vi "PSTR-Load Data.vi"(7 "selected path":path, 11 "error in (no error)":errorcluster, 12 "check":bool=TRUE) -> (4 "Params":T6={"Stimulus"={"Ear"=enum."Right", "BW (oct)"=0.3333, "Seed"=37, "Ramp (ms)"=1.0, "On time (ms)"=200.0, "Off time (ms)"=200.0, "Delay (ms)"=0.0}, "FreqSeq"={"Min (kHz)"=2.0, "Max (kHz)"=2.0, "Step (oct)"=0.5}, "LevelSeq"={"Min (dB)"=0.0, "Max (dB)"=80.0, "Step (dB)"=10.0}, "Seq"={"Order"=enum."Sequential", "Averages"=50}, "Response"={"Grass gain"=10000.0, "Window (ms)"=200.0}, "Hidden"={"Sample rate (Hz)"=100000.0, "Nfft"=2048, "save raw"=TRUE, "sep"=0.0, "Window"=enum."NONE"}, "RejThr"=0.0}, 6 "Data":T3, 8 "CFTS-PSTR":T2, 15 "error out":errorcluster)   [LabVIEW 2020]
uses:
  Typedefs/PSTR-Parameters.ctl
  Typedefs/PSTR-Stimulus Params.ctl
  epl-vi-lib/Utility VIs/Type Defs/Left-Right ring.ctl
  Typedefs/PSTR-FreqSeq Params.ctl
  Typedefs/PSTR-LevelSeq Params.ctl
  Typedefs/PSTR-SeqParams.ctl
  Typedefs/PSTR-Response Params.ctl
  Typedefs/PSTR-Hidden Params.ctl
  Typedefs/PSTR-Window Shape.ctl
  Typedefs/PSTR-Data.ctl
  Typedefs/PSTR-Model Fit.ctl
  Typedefs/PSTR-Fit Parameters.ctl
  Typedefs/PSTR-File Info.ctl
  <vilib>/regexp/Match Regular Expression.xnode
panel:
  in  "Data":T1
  # "NF x NL x 2 x Npts"
  # "NF x NL x Npts"
  # "NF x NL"
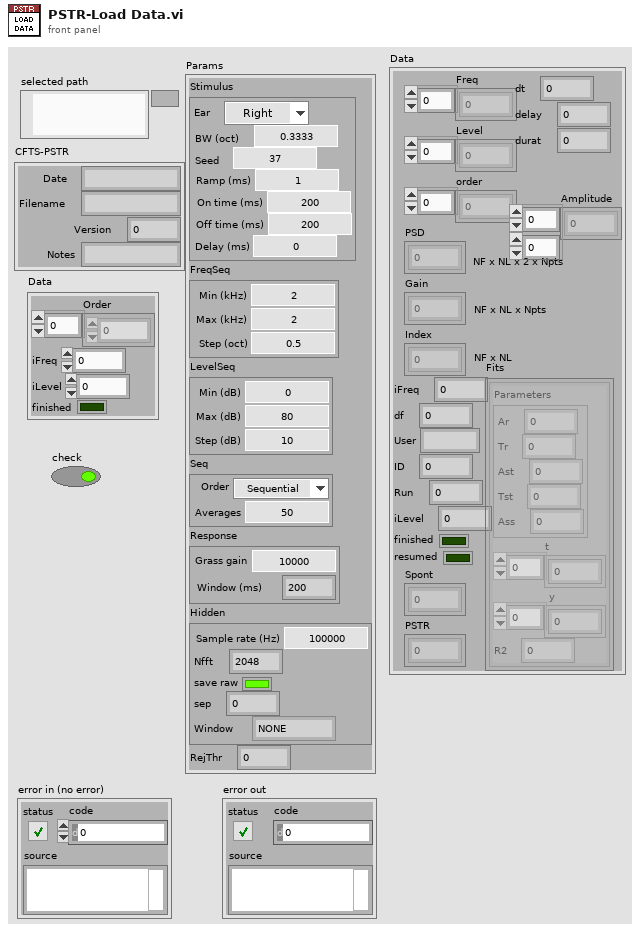
[diagram p1: front panel]
types:
  T1 = cluster{"Order":i32[], "iFreq":i32, "iLevel":i32, "finished":bool}
  T2 = typedef "PSTR-File Info.ctl" = cluster{"Date":string, "Filename":string, "Version":i32, "Notes":string}
  T3 = typedef "PSTR-Data.ctl" = cluster{"Freq":dbl[], "Level":dbl[], "order":i32[], "PSD":dbl[][][][], "Gain":dbl[][][], "Index":dbl[][], "iFreq":i32, "df":dbl, "User":string, "ID":i32, "Run":i32, "iLevel":i32, "finished":bool, "resumed":bool, "Spont":dbl[][], "PSTR":dbl[][][], "dt":dbl, "delay":dbl, "durat":dbl, "Fits":T4[][], "Amplitude":dbl[][]}
  T4 = typedef "PSTR-Model Fit.ctl" = cluster{"Parameters":T5, "t":dbl[], "y":dbl[], "R2":dbl}
  T5 = typedef "PSTR-Fit Parameters.ctl" = cluster{"Ar":dbl, "Tr":dbl, "Ast":dbl, "Tst":dbl, "Ass":dbl}
  T6 = typedef "PSTR-Parameters.ctl" = cluster{"Stimulus":T7, "FreqSeq":T9, "LevelSeq":T10, "Seq":T11, "Response":T12, "Hidden":T13, "RejThr":dbl}
  T7 = typedef "PSTR-Stimulus Params.ctl" = cluster{"Ear":T8, "BW (oct)":dbl, "Seed":i32, "Ramp (ms)":dbl, "On time (ms)":dbl, "Off time (ms)":dbl, "Delay (ms)":dbl}
  T8 = typedef "Left-Right ring.ctl" = enum16{"Right", "Left"}
  T9 = typedef "PSTR-FreqSeq Params.ctl" = cluster{"Min (kHz)":dbl, "Max (kHz)":dbl, "Step (oct)":dbl}
  T10 = typedef "PSTR-LevelSeq Params.ctl" = cluster{"Min (dB)":dbl, "Max (dB)":dbl, "Step (dB)":dbl}
  T11 = typedef "PSTR-SeqParams.ctl" = cluster{"Order":enum16{"Sequential", "Random"}, "Averages":i32}
  T12 = typedef "PSTR-Response Params.ctl" = cluster{"Grass gain":dbl, "Window (ms)":dbl}
  T13 = typedef "PSTR-Hidden Params.ctl" = cluster{"Sample rate (Hz)":dbl, "Nfft":i32, "save raw":bool, "sep":dbl, "Window":T14}
  T14 = typedef "PSTR-Window Shape.ctl" = enum16{"NONE", "Hamming"}
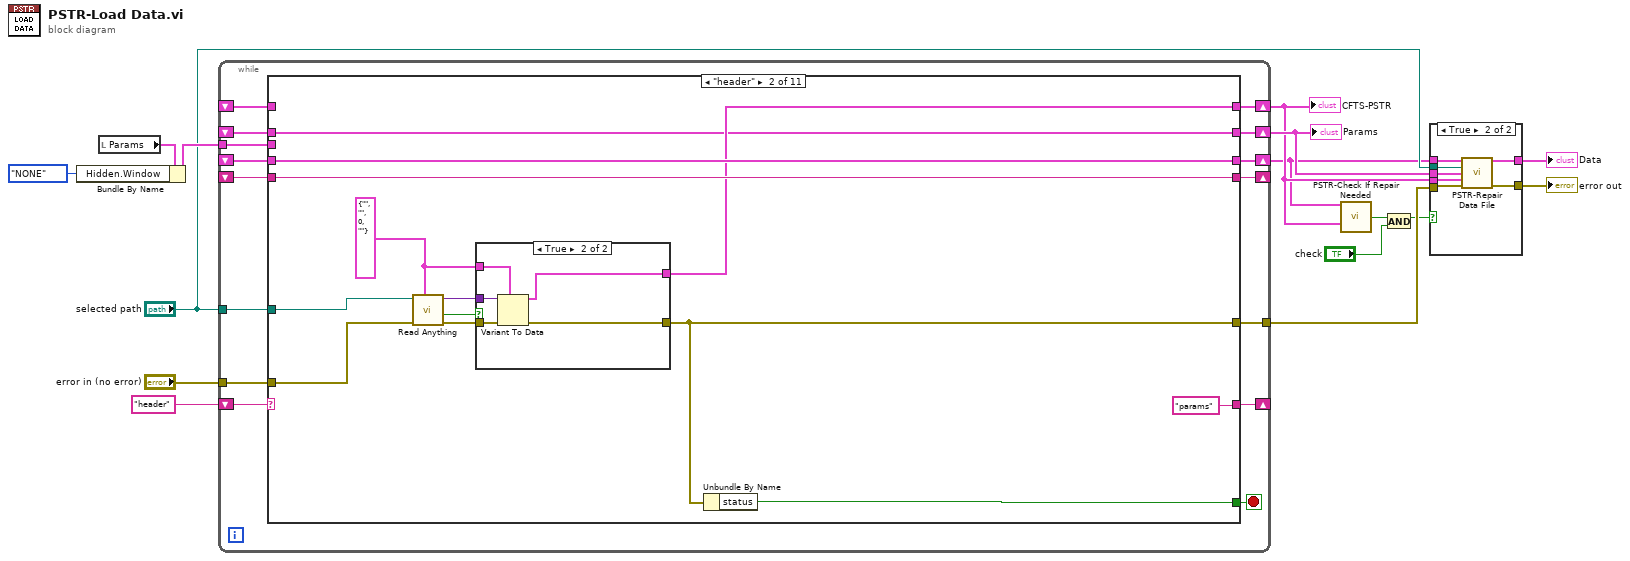
[diagram p0: block diagram]
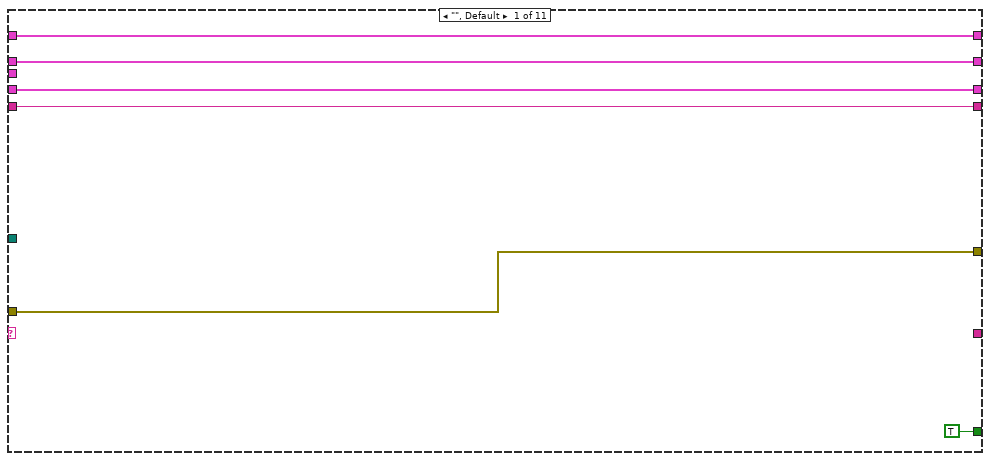
[diagram p2: hidden frame]
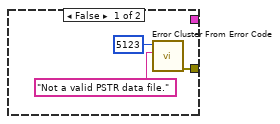
[diagram p3: hidden frame]
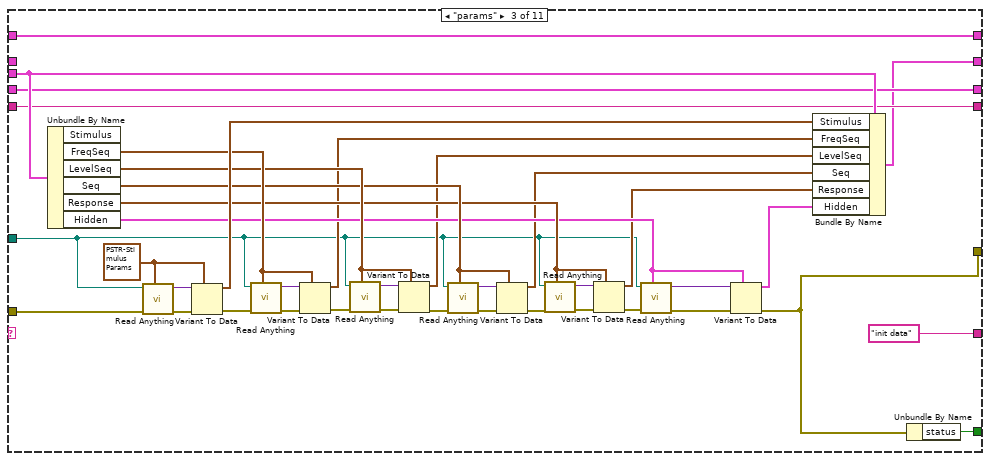
[diagram p4: hidden frame]
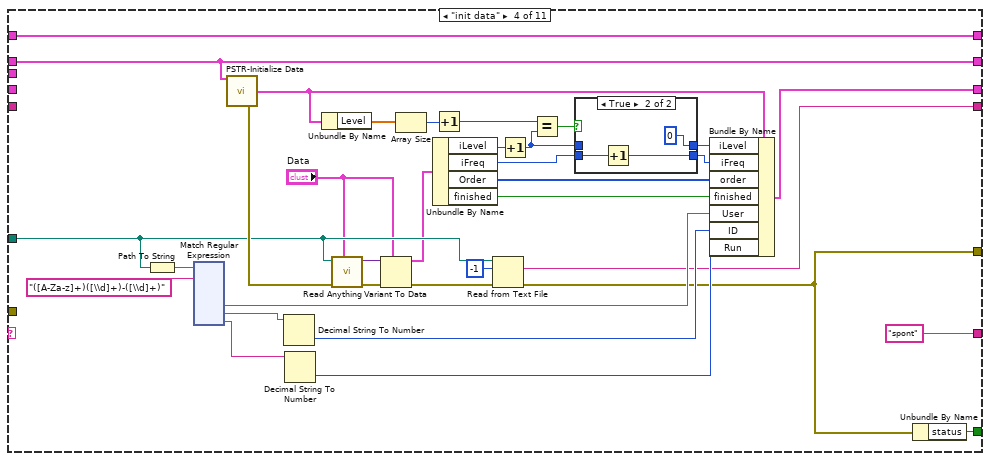
[diagram p5: hidden frame]
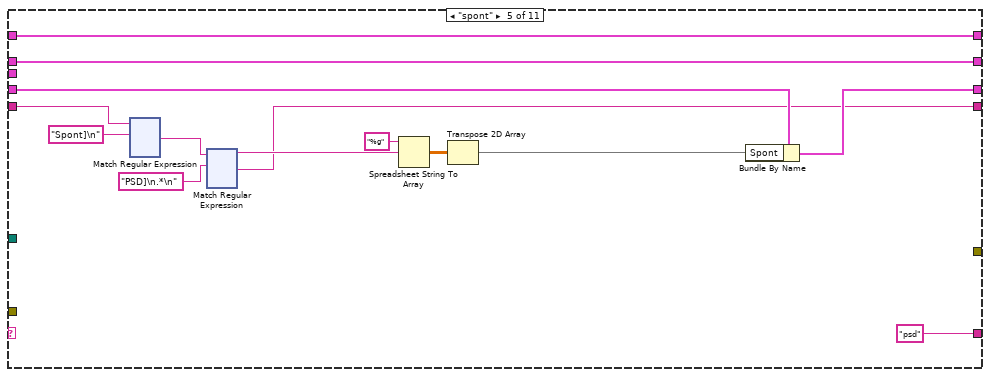
[diagram p7: hidden frame]
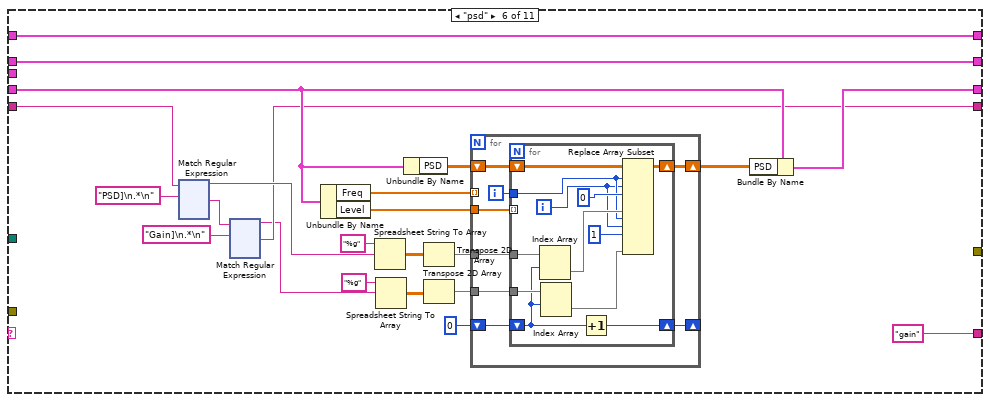
[diagram p8: hidden frame]
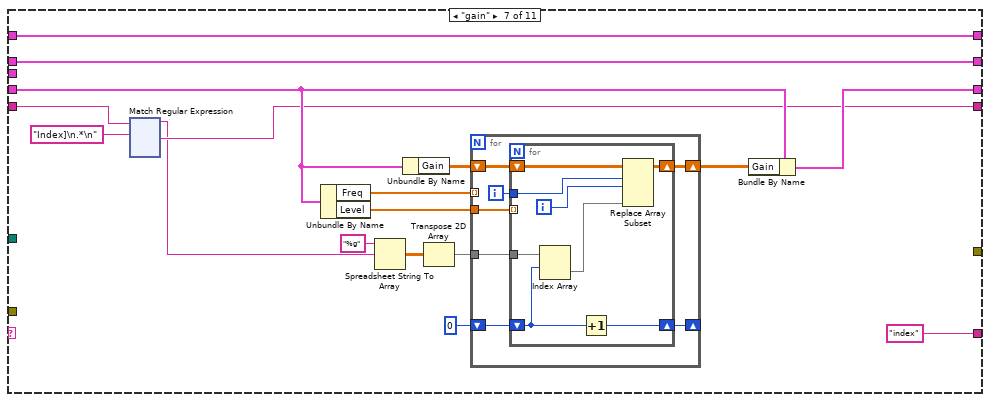
[diagram p9: hidden frame]
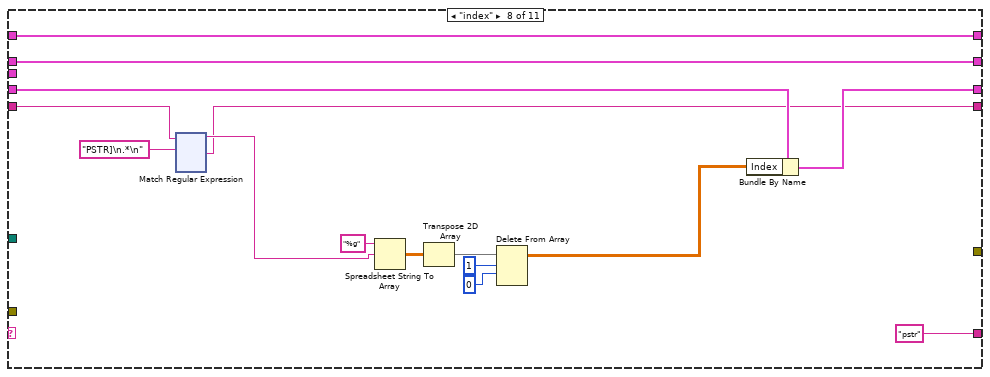
[diagram p10: hidden frame]
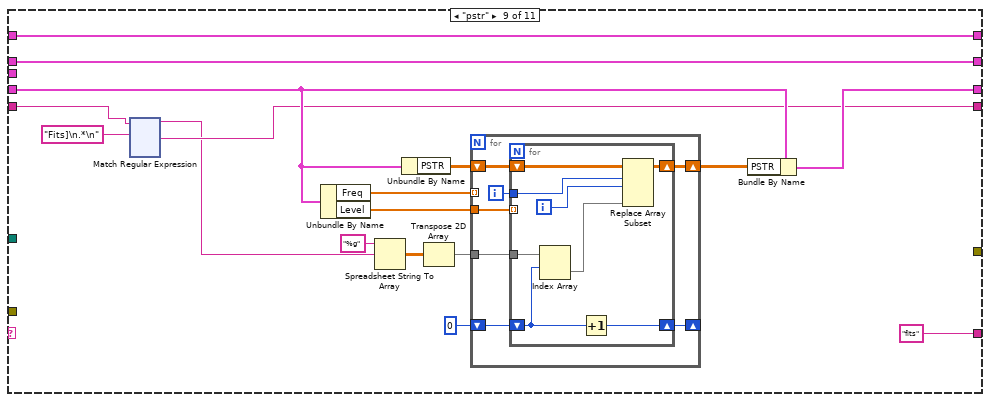
[diagram p11: hidden frame]
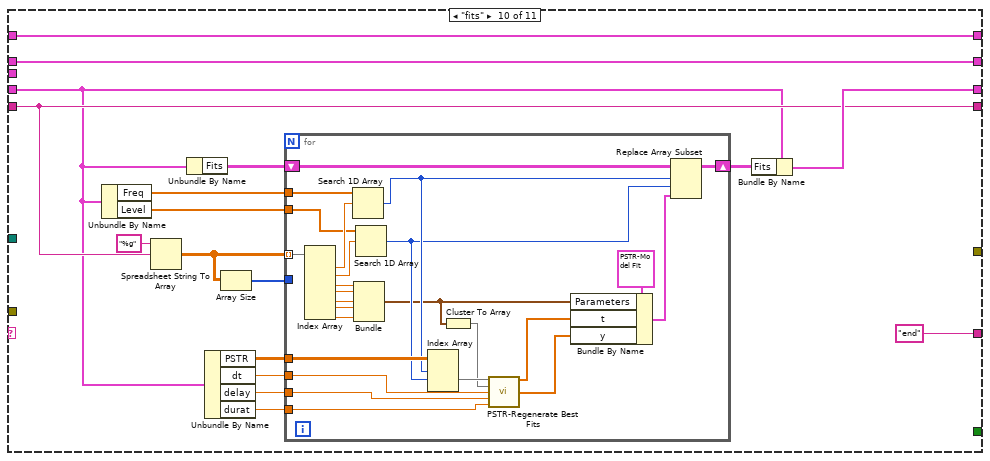
[diagram p12: hidden frame]
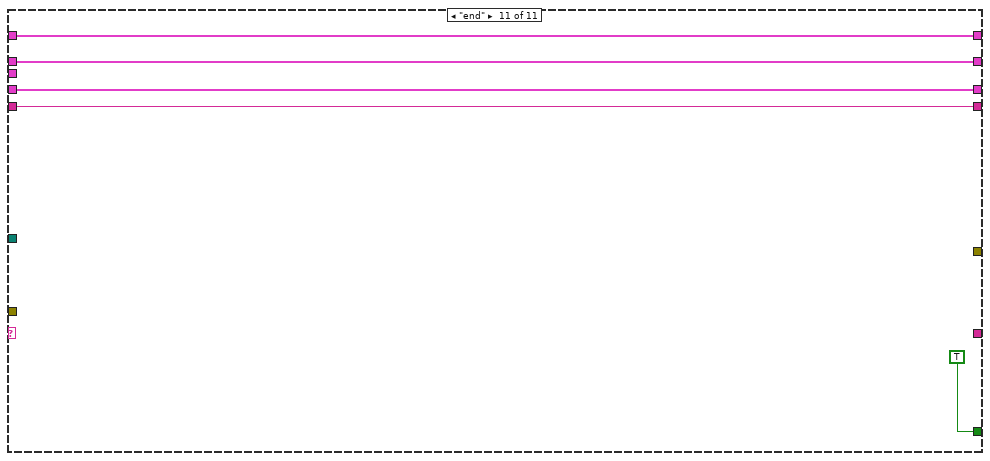
[diagram p13: hidden frame]
diagram:
  n1 = local read "Params"() -> (w13:T6)
  n2 = Bundle By Name(cluster=w13, "Hidden.Window"=PSTR-Window_Shape."NONE") -> (w12:T6)
  n3 = while {
    tunnel: "error in (no error)" -> [w30]
    tunnel: "selected path" -> [w29]
    shift-right: [w26] -> _
    shift-left: "header" -> [w28]
    tunnel: [w25] -> w3
    tunnel: w12 -> [w24]
    shift-right: [w23] -> w5
    shift-left: _ -> [w22]
    shift-right: [w21] -> _
    shift-left: _ -> [w20]
    shift-right: [w19] -> w6
    shift-left: _ -> [w18]
    shift-right: [w17] -> w8
    shift-left: _ -> [w16]
    stop <- w27 stop-if-true
    n4 = case shown="\"header\"" w28 {
      tunnel: w30 -> [w36 w49 w96 _ _ _ _ _ _ _ _]
      tunnel: w29 -> [_ w48 w63 w117 _ _ _ _ _ _ _]
      tunnel: [TRUE ("status") w42 w70 w126 _ _ _ _ _ _ TRUE ("status")] -> w27
      tunnel: [w36 w43 w71 w115 _ _ _ _ _ _ _] -> w25
      tunnel: [_ "params" "init data" "spont" "psd" "gain" "index" "pstr" "fits" "end" _] -> w26
      tunnel: w24 -> [_ _ w93 _ _ _ _ _ _ _ _]
      tunnel: [w34 w41 w62 w112 w265 w512 w777 w926 w1052 w1204 w1233] -> w23
      tunnel: w22 -> [w34 w41 w62 _ w266 w513 w778 w927 w1053 w1196 w1233]
      tunnel: [w33 w40 w61 w114 w256 w501 w770 w915 w1046 w1201 w1234] -> w21
      tunnel: w20 -> [w33 w40 w61 _ w263 w498 w773 w917 w1044 w1201 w1234]
      tunnel: [w32 w39 w59 w98 w255 w497 w768 w914 w1043 w1189 w1231] -> w19
      tunnel: w18 -> [w32 _ w59 w98 w255 w497 w768 w914 w1043 w1189 w1231]
      tunnel: [w31 w38 w58 w97 w254 w496 w767 w913 w1042 w1188 w1230] -> w17
      tunnel: w16 -> [w31 w38 _ w97 w254 w496 w767 w913 w1042 w1188 w1230]
      frame "", Default {
      }
      frame "header" {
        w37 = T2 {"Date"="", "Filename"="", "Version"=0, "Notes"=""} ("CFTS-PSTR")
        n5 = call "Read Anything.vi"("Type of Anything"=w37, "Error In"=w49, "Path (dialog)"=w48) -> ("Error Out"=w47:errorcluster, "Found?"=w46:bool, "Anything"=w45:variant)  [unwired: 6 in]
        n6 = case shown="True" w46 {
          tunnel: w47 -> [_ w57]
          tunnel: w45 -> [_ w56]
          tunnel: w37 -> [_ w55]
          tunnel: [w52 w54] -> w43
          tunnel: [_ w53] -> w39
          frame False {
            n7 = call <vilib>:"Error Cluster From Error Code.vi"("error message (\"\")"="Not a valid PSTR data file." ("error message (\"\")"), "error code (0)"=5123) -> ("error out"=w52:errorcluster)  [unwired: 7 in]
          }
          frame True {
            n8 = Variant To Data(error in=w57, type=w55, Variant=w56) -> (data=w53:T2, error out=w54:errorcluster)
          }
        }
        n9 = Unbundle By Name(w43) -> ("status"=w42:bool)
      }
      frame "params" {
        w60 = T7 {"Ear"=enum."Right", "BW (oct)"=0.25, "Seed"=37, "Ramp (ms)"=5.0, "On time (ms)"=300.0, "Off time (ms)"=300.0, "Delay (ms)"=0.0} ("Stimulus")
        n10 = Unbundle By Name(w93) -> ("FreqSeq"=w88:T9, "LevelSeq"=w84:T10, "Seq"=w74:T11, "Response"=w73:T12, "Hidden"=w72:T13)  [unwired: 1 out]
        n11 = call "Read Anything.vi"("Type of Anything"=w60, "Error In"=w96, "Path (dialog)"=w63) -> ("Error Out"=w95:errorcluster, "Anything"=w94:variant)  [unwired: 6 in, 1 out]
        n12 = Variant To Data(error in=w95, type=w60, Variant=w94) -> (data=w92:T7, error out=w89:errorcluster)
        n13 = call "Read Anything.vi"("Type of Anything"=w88, "Error In"=w89, "Path (dialog)"=w63) -> ("Error Out"=w91:errorcluster, "Anything"=w90:variant)  [unwired: 6 in, 1 out]
        n14 = Variant To Data(error in=w91, type=w88, Variant=w90) -> (data=w68:T9, error out=w86:errorcluster)
        n15 = call "Read Anything.vi"("Type of Anything"=w84, "Error In"=w86, "Path (dialog)"=w63) -> ("Error Out"=w87:errorcluster, "Anything"=w85:variant)  [unwired: 6 in, 1 out]
        n16 = Variant To Data(error in=w87, type=w84, Variant=w85) -> (data=w67:T10, error out=w77:errorcluster)
        n17 = call "Read Anything.vi"("Type of Anything"=w74, "Error In"=w77, "Path (dialog)"=w63) -> ("Error Out"=w83:errorcluster, "Anything"=w82:variant)  [unwired: 6 in, 1 out]
        n18 = Variant To Data(error in=w83, type=w74, Variant=w82) -> (data=w66:T11, error out=w76:errorcluster)
        n19 = call "Read Anything.vi"("Type of Anything"=w73, "Error In"=w76, "Path (dialog)"=w63) -> ("Error Out"=w81:errorcluster, "Anything"=w80:variant)  [unwired: 6 in, 1 out]
        n20 = Variant To Data(error in=w81, type=w73, Variant=w80) -> (data=w65:T12, error out=w75:errorcluster)
        n21 = call "Read Anything.vi"("Type of Anything"=w72, "Error In"=w75, "Path (dialog)"=w63) -> ("Error Out"=w79:errorcluster, "Anything"=w78:variant)  [unwired: 6 in, 1 out]
        n22 = Variant To Data(error in=w79, type=w72, Variant=w78) -> (data=w64:T13, error out=w71:errorcluster)
        n23 = Bundle By Name(cluster=w93, "Stimulus"=w92, "FreqSeq"=w68, "LevelSeq"=w67, "Seq"=w66, "Response"=w65, "Hidden"=w64) -> (w58:T6)
        n24 = Unbundle By Name(w71) -> ("status"=w70:bool)
      }
      frame "init data" {
        n25 = Path To String(path=w117) -> (string=w125:string)
        n26 = xnode "Match Regular Expression"("input string"=w125, "regular expression"="([A-Za-z]+)([\\d]+)-([\\d]+)") -> ("submatch 1"=w123:string, "submatch 2"=w122:string, "submatch 3"=w120:string)  [unwired: 4 in, 5 out]
        n27 = call "PSTR-Initialize Data.vi"("PSTR Params"=w97) -> ("Data"=w109:T3, "error out"=w128:errorcluster)  [unwired: 13 in]
        n28 = Decimal String To Number(string=w122) -> (number=w121:i32)  [unwired: 2 in, 1 out]
        n29 = Decimal String To Number(string=w120) -> (number=w119:i32)  [unwired: 2 in, 1 out]
        n30 = Unbundle By Name(w109) -> ("Level"=w108:dbl[])
        n31 = call "Read Anything.vi"("Type of Anything"="Data", "Error In"=w128, "Path (dialog)"=w117) -> ("Error Out"=w130:errorcluster, "Anything"=w129:variant)  [unwired: 6 in, 1 out]
        n32 = Variant To Data(error in=w130, type="Data", Variant=w129) -> (data=w113:T1, error out=w118:errorcluster)
        n33 = Array Size(array=w108) -> (size(s)=w107:i32)
        n34 = Unbundle By Name(w113) -> ("iLevel"=w110:i32, "iFreq"=w104:i32, "Order"=w105:i32[], "finished"=w99:bool)
        n35 = Increment(x=w107) -> (x+1=w102:i32)
        n36 = Read from Text File(file (use dialog)=w117, count=-1, error in=w118) -> (text=w114:string, error out=w115:errorcluster)  [unwired: 1 in, 2 out]
        n37 = Increment(x=w110) -> (x+1=w100:i32)
        n38 = Equal?(x=w102, y=w100) -> (x = y?=w106:bool)
        n39 = case shown="True" w106 {
          tunnel: w104 -> [w132 w135]
          tunnel: [w132 w134] -> w103
          tunnel: [w131 0] -> w101
          tunnel: w100 -> [w131 _]
          frame False {
          }
          frame True {
            n40 = Increment(x=w135) -> (x+1=w134:i32)
          }
        }
        n41 = Bundle By Name(cluster=w109, "iLevel"=w101, "iFreq"=w103, "order"=w105, "finished"=w99, "User"=w123, "ID"=w121, "Run"=w119) -> (w112:T3)
        n42 = Unbundle By Name(w115) -> ("status"=w126:bool)
      }
      frame "spont" {
        n43 = xnode "Match Regular Expression"("input string"=w263, "regular expression"="Spont]\n" ("search string/char (-)")) -> ("after match"=w259:string)  [unwired: 4 in, 4 out]
        n44 = xnode "Match Regular Expression"("input string"=w259, "regular expression"="PSD]\n.*\n" ("search string/char (-)")) -> ("before match"=w257:string, "after match"=w256:string)  [unwired: 4 in, 3 out]
        n45 = Spreadsheet String To Array(format string="%g", spreadsheet string=w257) -> (array=w267:dbl[][])  [unwired: 2 in]
        n46 = Transpose 2D Array(2D array=w267) -> (transposed array=w260:dbl[][])
        n47 = Bundle By Name(cluster=w266, "Spont"=w260) -> (w265:T3)
      }
      frame "psd" {
        n48 = xnode "Match Regular Expression"("input string"=w498, "regular expression"="PSD]\n.*\n" ("search string/char (-)")) -> ("before match"=w504:string, "after match"=w503:string)  [unwired: 4 in, 3 out]
        n49 = xnode "Match Regular Expression"("input string"=w503, "regular expression"="Gain]\n.*\n" ("search string/char (-)")) -> ("before match"=w500:string, "after match"=w501:string)  [unwired: 4 in, 3 out]
        n50 = Unbundle By Name(w513) -> ("Freq"=w515:dbl[], "Level"=w516:dbl[])
        n51 = Spreadsheet String To Array(format string="%g", spreadsheet string=w504) -> (array=w517:dbl[][])  [unwired: 2 in]
        n52 = Spreadsheet String To Array(format string="%g", spreadsheet string=w500) -> (array=w506:dbl[][])  [unwired: 2 in]
        n53 = Unbundle By Name(w513) -> ("PSD"=w518:dbl[][][][])
        n54 = Transpose 2D Array(2D array=w517) -> (transposed array=w509:dbl[][])
        n55 = Transpose 2D Array(2D array=w506) -> (transposed array=w505:dbl[][])
        n56 = for {
          shift-right: [w753] -> w514
          shift-left: w518 -> [w754]
          tunnel: w509 -> [w750]
          tunnel: w515 -> [_] mode=indexing
          tunnel: w516 -> [w751]
          shift-right: [w748] -> _
          shift-left: 0 -> [w749]
          tunnel: w505 -> [w747]
          i -> [w752]
          n57 = for {
            shift-right: [w765] -> w753
            shift-left: w754 -> [w766]
            tunnel: w752 -> [w758]
            tunnel: w751 -> [_] mode=indexing
            tunnel: w750 -> [w762]
            shift-right: [w763] -> w748
            shift-left: w749 -> [w759]
            tunnel: w747 -> [w760]
            i -> [w757]
            n58 = Index Array(array=w762, index (row)=w759) -> (element=w761:dbl[])  [unwired: 1 in]
            n59 = Index Array(array=w760, index (row)=w759) -> (element=w755:dbl[])  [unwired: 1 in]
            n60 = Increment(x=w759) -> (x+1=w763:i32)
            n61 = Replace Array Subset(array=w766, new element #1=w761, index (dim 0) #1=w758, index (dim 1) #1=w757, index (dim 2) #1=0 ("disabled index (row)"), new element #2=w755, index (dim 0) #2=w758, index (dim 1) #2=w757, index (dim 2) #2=1 ("disabled index (row)")) -> (w765:dbl[][][][])  [unwired: 2 in]
          }
        }
        n62 = Bundle By Name(cluster=w513, "PSD"=w514) -> (w512:T3)
      }
      frame "gain" {
        n63 = xnode "Match Regular Expression"("input string"=w773, "regular expression"="Index]\n.*\n" ("search string/char (-)")) -> ("before match"=w769:string, "after match"=w770:string)  [unwired: 4 in, 3 out]
        n64 = Unbundle By Name(w778) -> ("Freq"=w780:dbl[], "Level"=w781:dbl[])
        n65 = Spreadsheet String To Array(format string="%g", spreadsheet string=w769) -> (array=w782:dbl[][])  [unwired: 2 in]
        n66 = Unbundle By Name(w778) -> ("Gain"=w783:dbl[][][])
        n67 = Transpose 2D Array(2D array=w782) -> (transposed array=w774:dbl[][])
        n68 = for {
          shift-right: [w903] -> w779
          shift-left: w783 -> [w904]
          tunnel: w774 -> [w900]
          tunnel: w780 -> [_] mode=indexing
          tunnel: w781 -> [w901]
          shift-right: [w898] -> _
          shift-left: 0 -> [w899]
          i -> [w902]
          n69 = for {
            shift-right: [w911] -> w903
            shift-left: w904 -> [w912]
            tunnel: w902 -> [w906]
            tunnel: w901 -> [_] mode=indexing
            tunnel: w900 -> [w909]
            shift-right: [w910] -> w898
            shift-left: w899 -> [w907]
            i -> [w905]
            n70 = Index Array(array=w909, index (row)=w907) -> (element=w908:dbl[])  [unwired: 1 in]
            n71 = Increment(x=w907) -> (x+1=w910:i32)
            n72 = Replace Array Subset(array=w912, new element=w908, index (dim 0)=w906, index (dim 1)=w905) -> (w911:dbl[][][])  [unwired: 1 in]
          }
        }
        n73 = Bundle By Name(cluster=w778, "Gain"=w779) -> (w777:T3)
      }
      frame "index" {
        n74 = xnode "Match Regular Expression"("input string"=w917, "regular expression"="PSTR]\n.*\n" ("search string/char (-)")) -> ("before match"=w916:string, "after match"=w915:string)  [unwired: 4 in, 3 out]
        n75 = Spreadsheet String To Array(format string="%g", spreadsheet string=w916) -> (array=w924:dbl[][])  [unwired: 2 in]
        n76 = Transpose 2D Array(2D array=w924) -> (transposed array=w922:dbl[][])
        n77 = Delete From Array(array=w922, length=1, index (row)=0) -> (array with subset deleted=w919:dbl[][])  [unwired: 1 in, 1 out]
        n78 = Bundle By Name(cluster=w927, "Index"=w919) -> (w926:T3)
      }
      frame "pstr" {
        n79 = xnode "Match Regular Expression"("input string"=w1044, "regular expression"="Fits]\n.*\n" ("search string/char (-)")) -> ("before match"=w1045:string, "after match"=w1046:string)  [unwired: 4 in, 3 out]
        n80 = Unbundle By Name(w1053) -> ("Freq"=w1055:dbl[], "Level"=w1056:dbl[])
        n81 = Spreadsheet String To Array(format string="%g", spreadsheet string=w1045) -> (array=w1057:dbl[][])  [unwired: 2 in]
        n82 = Unbundle By Name(w1053) -> ("PSTR"=w1058:dbl[][][])
        n83 = Transpose 2D Array(2D array=w1057) -> (transposed array=w1049:dbl[][])
        n84 = for {
          shift-right: [w1178] -> w1054
          shift-left: w1058 -> [w1179]
          tunnel: w1049 -> [w1175]
          tunnel: w1055 -> [_] mode=indexing
          tunnel: w1056 -> [w1176]
          shift-right: [w1173] -> _
          shift-left: 0 -> [w1174]
          i -> [w1177]
          n85 = for {
            shift-right: [w1186] -> w1178
            shift-left: w1179 -> [w1187]
            tunnel: w1177 -> [w1181]
            tunnel: w1176 -> [_] mode=indexing
            tunnel: w1175 -> [w1184]
            shift-right: [w1185] -> w1173
            shift-left: w1174 -> [w1182]
            i -> [w1180]
            n86 = Index Array(array=w1184, index (row)=w1182) -> (element=w1183:dbl[])  [unwired: 1 in]
            n87 = Increment(x=w1182) -> (x+1=w1185:i32)
            n88 = Replace Array Subset(array=w1187, new element=w1183, index (dim 0)=w1181, index (dim 1)=w1180) -> (w1186:dbl[][][])  [unwired: 1 in]
          }
        }
        n89 = Bundle By Name(cluster=w1053, "PSTR"=w1054) -> (w1052:T3)
      }
      frame "fits" {
        n90 = Unbundle By Name(w1196) -> ("Freq"=w1198:dbl[], "Level"=w1199:dbl[])
        n91 = Spreadsheet String To Array(format string="%g", spreadsheet string=w1201) -> (array=w1191:dbl[][])  [unwired: 2 in]
        n92 = Unbundle By Name(w1196) -> ("Fits"=w1200:T4[][])
        n93 = Unbundle By Name(w1196) -> ("PSTR"=w1195:dbl[][][], "dt"=w1194:dbl, "delay"=w1193:dbl, "durat"=w1192:dbl)
        n94 = Array Size(array=w1191) -> (size(s)=w1190:i32[])
        n95 = for {
          shift-right: [w1228] -> w1197
          shift-left: w1200 -> [w1229]
          tunnel: w1191 -> [w1227] mode=indexing
          tunnel: w1198 -> [w1226]
          tunnel: w1199 -> [w1224]
          tunnel: w1195 -> [w1215]
          tunnel: w1194 -> [w1211]
          tunnel: w1193 -> [w1210]
          tunnel: w1192 -> [w1209]
          tunnel: w1190 -> [_]
          n96 = Index Array(array=w1227) -> (element #1=w1225:dbl, element #2=w1223:dbl, element #3=w1222:dbl, element #4=w1221:dbl, element #5=w1220:dbl, element #6=w1219:dbl, element #7=w1218:dbl)  [unwired: 7 in]
          n97 = Search 1D Array(1D array=w1226, element=w1225) -> (index of element=w1214:i32)  [unwired: 1 in]
          n98 = Bundle(w1222, w1221, w1220, w1219, w1218) -> (w1208:cluster{dbl, dbl, dbl, dbl, dbl})  [unwired: 1 in]
          n99 = Search 1D Array(1D array=w1224, element=w1223) -> (index of element=w1213:i32)  [unwired: 1 in]
          n100 = Index Array(array=w1215, index (dim 0)=w1214, index (dim 1)=w1213) -> (element=w1212:dbl[])  [unwired: 1 in]
          n101 = Cluster To Array(cluster=w1208) -> (array=w1207:dbl[])
          n102 = call "PSTR-Regenerate Best Fits.vi"("PSTH"=w1212, "params"=w1207, "dt (ms)"=w1211, "delay (ms)"=w1210, "durat (ms)"=w1209) -> ("t"=w1206:dbl[], "y"=w1205:dbl[])  [unwired: 9 in]
          n103 = Bundle By Name(cluster=T4 {"Parameters"={"Ar"=0.0, "Tr"=0.0, "Ast"=0.0, "Tst"=0.0, "Ass"=0.0}, "t"=[], "y"=[], "R2"=0.0} ("new element/subarray"), "Parameters"=w1208, "t"=w1206, "y"=w1205) -> (w1216:T4)
          n104 = Replace Array Subset(array=w1229, new element=w1216, index (row)=w1214, index (col)=w1213) -> (w1228:T4[][])
        }
        n105 = Bundle By Name(cluster=w1196, "Fits"=w1197) -> (w1204:T3)
      }
      frame "end" {
      }
    }
  }
  "CFTS-PSTR" <- w6
  "Params" <- w8
  n106 = call "PSTR-Check If Repair Needed.vi"("Data in"=w5, "CFTS-PSTR"=w6) -> ("needs repair"=w4:bool)  [unwired: 13 in]
  n107 = And(x=w4, y="check") -> (x .and. y?=w2:bool)
  n108 = case shown="True" w2 {
    tunnel: w5 -> [w1236 w1242]
    tunnel: [w1236 w1243] -> w10
    tunnel: "selected path" -> [_ w1241]
    tunnel: w6 -> [_ w1240]
    tunnel: w8 -> [_ w1239]
    tunnel: w3 -> [w1235 w1238]
    tunnel: [w1235 w1237] -> w7
    frame False {
    }
    frame True {
      n109 = call "PSTR-Repair Data File.vi"("Data in"=w1242, "path"=w1241, "PSTR Params"=w1239, "CFTS-PSTR"=w1240, "error in (no error)"=w1238) -> ("Data out"=w1243:T3, "error out"=w1237:errorcluster)  [unwired: 9 in]
    }
  }
  "error out" <- w7
  "Data" <- w10
